vi "MatchPiezoLaserSignals.vi"(6 "Use 1 frame for this laser Channel":bool, 8 "LaserSigIn":dbl[](array[numeric]), 9 "VolumeNumberIn":dbl[](array[numeric]), 10 "PiezoSig":dbl[](array[numeric])) -> (1 "LaserSigOut":dbl[](array[numeric]), 2 "VolumeNumberOut":dbl[](array[numeric]), 3 "PiezoSigOut":dbl[](array[numeric]))   [LabVIEW 2015]
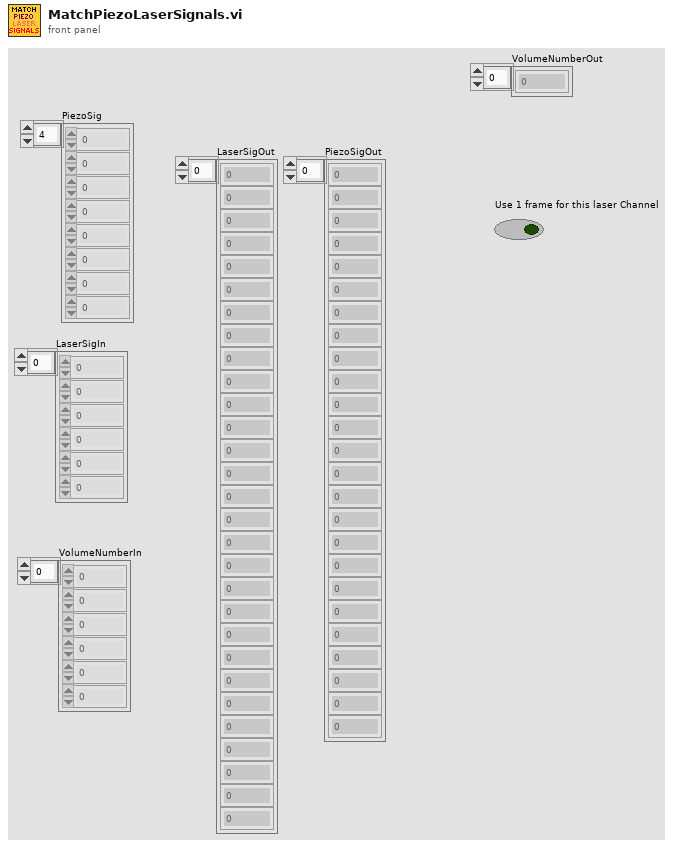
[diagram p1: front panel]
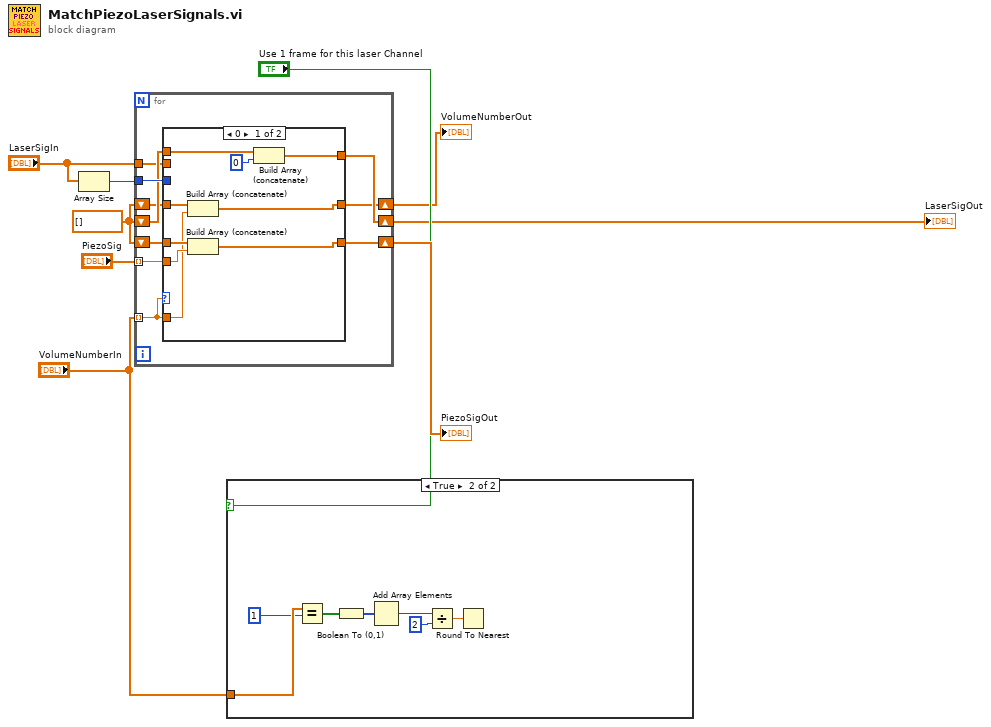
[diagram p0: block diagram]
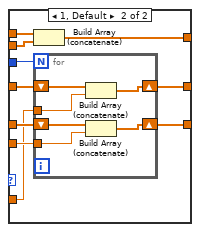
[diagram p3: hidden frame]
diagram:
  w5 = dbl[] [] ("appended array")
  n1 = Array Size(array="LaserSigIn") -> (size(s)=w8:i32)
  n2 = for {
    shift-right: [w15] -> w1
    shift-left: w5 -> [w14]
    tunnel: w8 -> [w19]
    tunnel: "PiezoSig" -> [w18] mode=indexing
    shift-right: [w16] -> w7
    shift-left: w5 -> [w17]
    tunnel: "LaserSigIn" -> [w13]
    tunnel: "VolumeNumberIn" -> [w11] mode=indexing
    shift-right: [w10] -> w2
    shift-left: w5 -> [w12]
    n3 = case shown="0" w11 {
      tunnel: w19 -> [_ w38]
      tunnel: w18 -> [w27 w37]
      tunnel: w17 -> [w28 w36]
      tunnel: [w26 w35] -> w16
      tunnel: [w23 w34] -> w15
      tunnel: w14 -> [w24 w33]
      tunnel: w13 -> [_ w32]
      tunnel: w12 -> [w22 w31]
      tunnel: w11 -> [w21 w30]
      tunnel: [w20 w29] -> w10
      frame 0 {
        n4 = Build Array (concatenate)(w22, w21) -> (w20:dbl[])
        n5 = Build Array (concatenate)(w28, w27) -> (w26:dbl[])
        n6 = Build Array (concatenate)(w24, 0) -> (w23:dbl[])
      }
      frame 1, Default {
        n7 = Build Array (concatenate)(w33, w32) -> (w34:dbl[])
        n8 = for {
          N: w38 -> [_]
          tunnel: w37 -> [w43]
          shift-right: [w42] -> w35
          shift-left: w36 -> [w44]
          shift-right: [w39] -> w29
          shift-left: w31 -> [w41]
          tunnel: w30 -> [w40]
          n9 = Build Array (concatenate)(w41, w40) -> (w39:dbl[])
          n10 = Build Array (concatenate)(w44, w43) -> (w42:dbl[])
        }
      }
    }
  }
  "LaserSigOut" <- w1
  "PiezoSigOut" <- w7
  "VolumeNumberOut" <- w2
  n11 = case shown="True" "Use 1 frame for this laser Channel" {
    tunnel: "VolumeNumberIn" -> [_ w46]
    frame False {
    }
    frame True {
      n12 = Equal?(x=w46, y=i16 1) -> (x = y?=w51:bool[])
      n13 = Boolean To (0,1)(Boolean=w51) -> (0, 1=w50:i16[])
      n14 = Add Array Elements(numeric array=w50) -> (sum=w49:i16)
      n15 = Divide(x=w49, y=i16 2) -> (x/y=w47:dbl)
      n16 = Round To Nearest(number=w47) -> ()  [unwired: 1 out]
    }
  }
